vi "Convert C to F.vi"(1 "섭씨":dbl) -> (0 "화씨":dbl)   [LabVIEW 2010]
doc: "이 VI는 섭씨로 읽은 값을 화씨로 변환합니다."
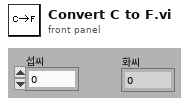
[diagram p1: front panel]
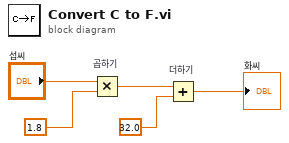
[diagram p0: block diagram]
diagram:
  n1 = Multiply "곱하기"(x="섭씨", y=1.8) -> (x*y=w3:dbl)
  n2 = Add "더하기"(x=w3, y=32.0) -> (x+y=→"화씨":dbl)
